vi "MainForceMeasurement.vi"() -> ()   [LabVIEW 2010]
uses:
  <vilib>/Instr/_visa.llb/VISA Flush IO Buffer Mask.ctl
  Variable globale 1.vi
  <vilib>/Instr/_visa.llb/VISA Configure Serial Port (Instr).vi
panel:
  out "Data":dbl[](array[numeric])
  out "Waveform Chart":dynamicdata(graph)
  in  "attente (ms)":u32=50
  in  "Temps échelon":i32=25
  out "Sor":string[][](array[string]) caption="Motor torque"
  out "Ent":string[][](array[string]) caption="Motor commande"
  out "Con_XYLeftTorque 2":cluster{"Y":dbl[], "Y":dbl[]}[](graph) caption="Sortie"
  out "Con_XYLeftTorque":cluster{"Y":dbl[], "Y":dbl[]}[](graph) caption="Commande"
  in  "Temps départ":i32=25
  out "tableau inversé 2":u8[](array[numeric])
  out "tableau inversé":i8[](array[numeric])
  out "error out 2":errorcluster caption="sortie d'erreur"
  in  "Type moteur":i32=139 min=0 max=255
  out "Float recu":sgl
  in  "Couple":sgl=25.45
  out "Iteration 3":i32
  out "Iteration reception":i32
  out "Iteration Envoi":i32
  out "Checksum calculé":i32
  out "Checksum reçu":i32
  out "Type de donnee (ID)":i32
  out "Byte Start ?":bool
  out "Retour 2":string
  in  "stop secu":bool
  in  "STOP":bool
  out "error out":errorcluster caption="sortie d'erreur"
  in  "baud rate (9600)":u32=9600 caption="débit en bauds (9600)"
  in  "Port Com":refnum<visa-resource-name>="COM7" caption="Nom de ressource VISA"
  # "Paramètre de l'envoi de l'échelon"
  # "Réception"
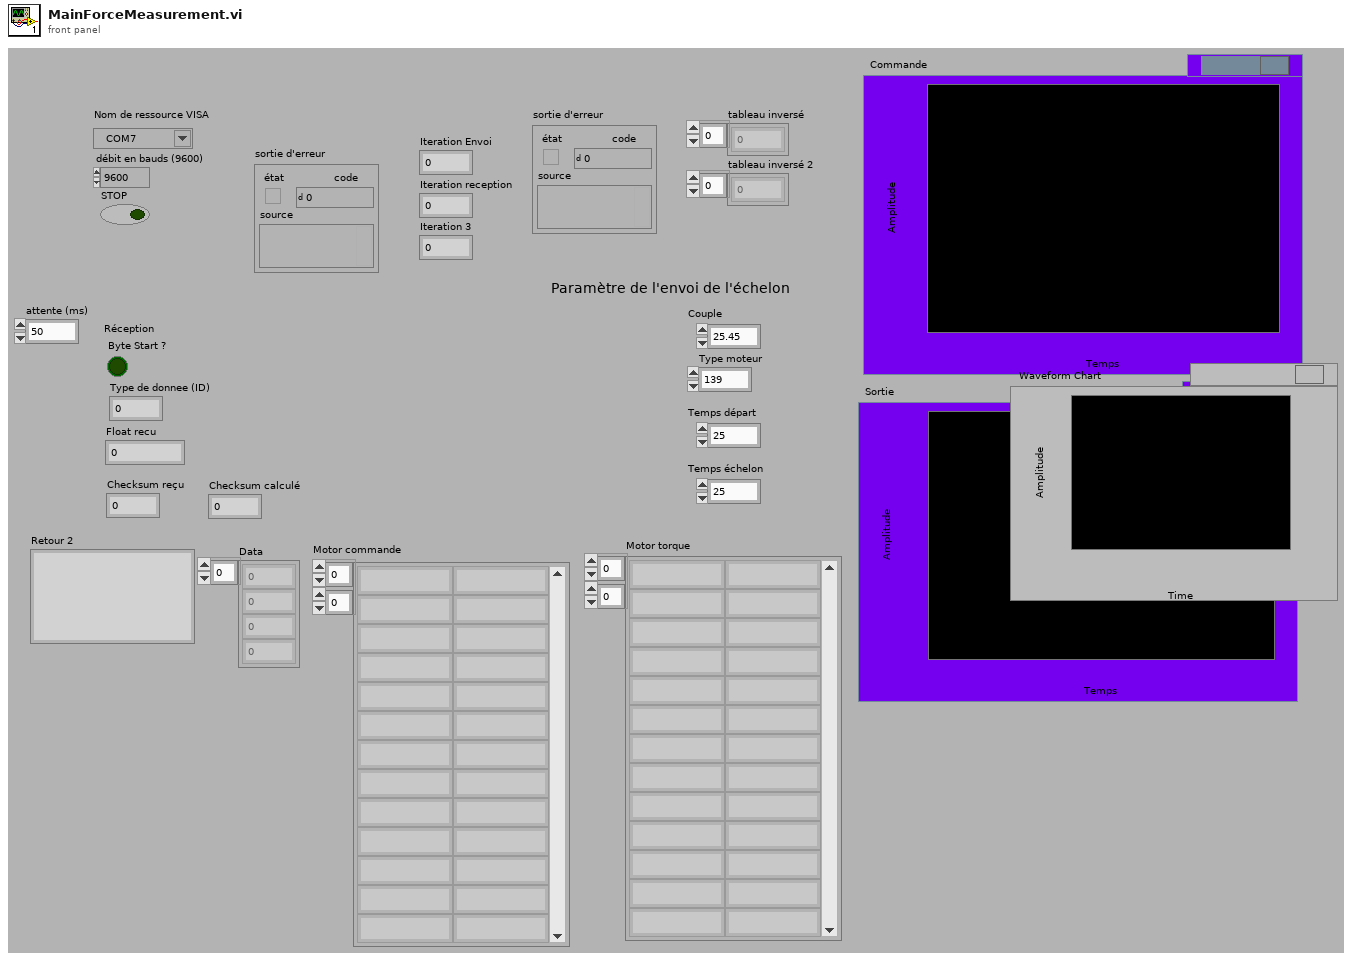
[diagram p1: front panel]
types:
  T1 = typedef "VISA Flush IO Buffer Mask.ctl" = u16
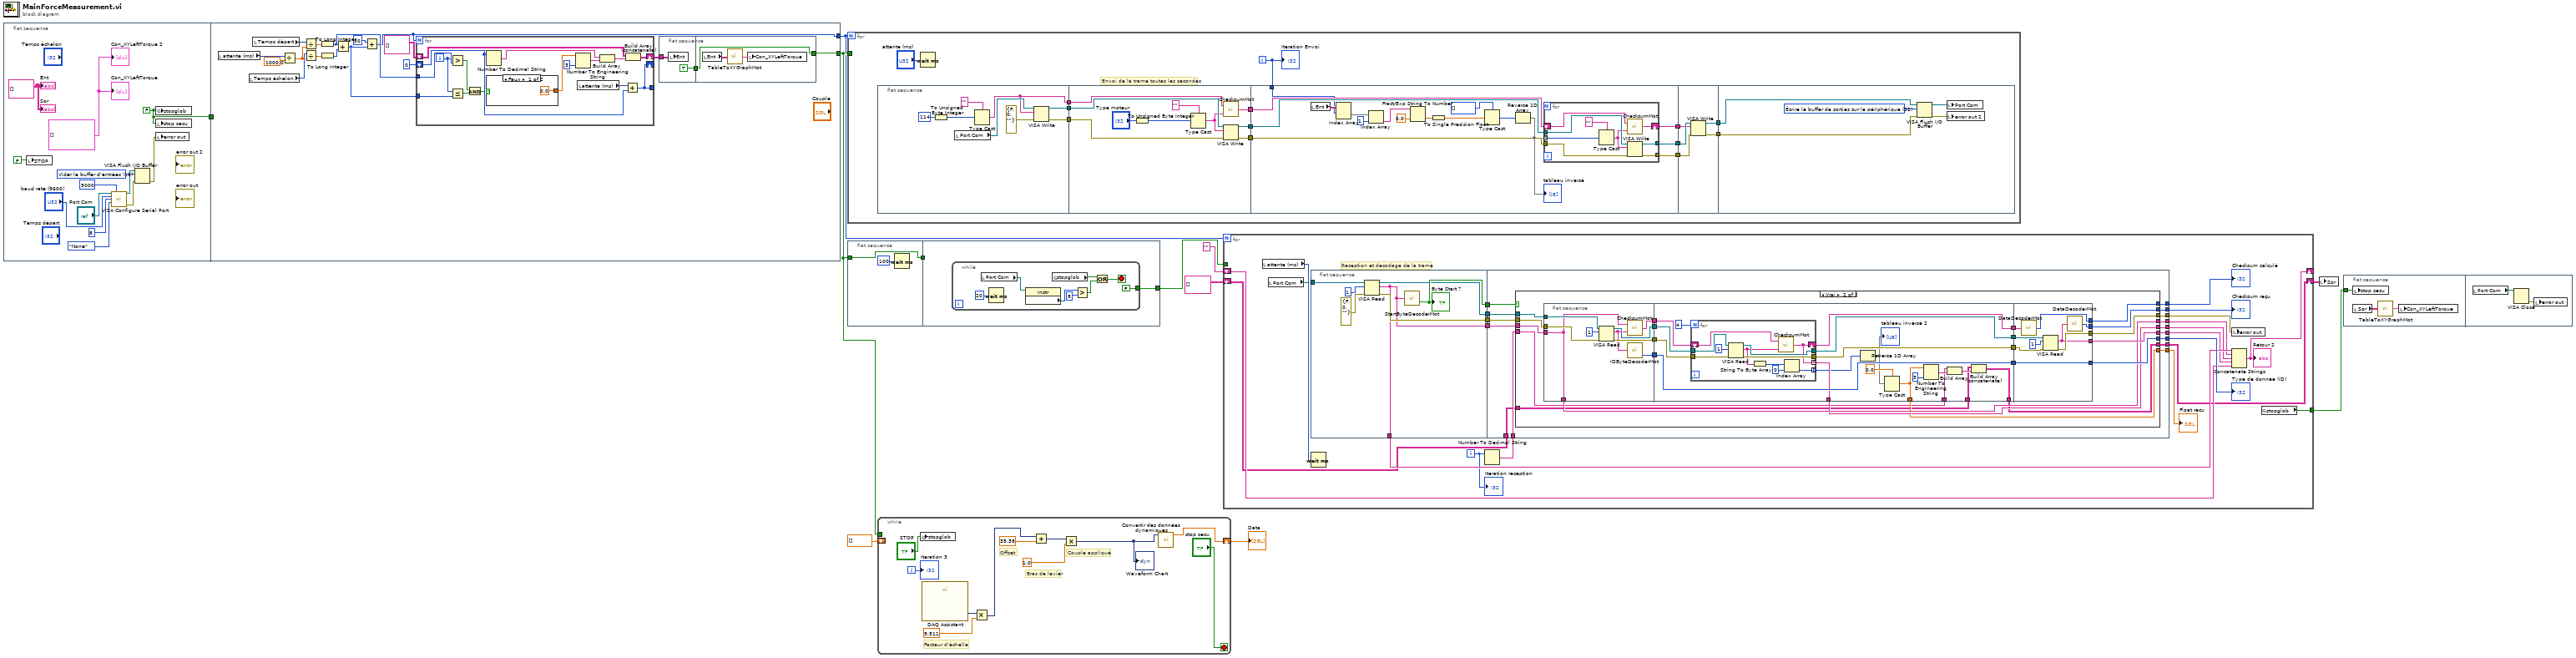
[diagram p0: block diagram]
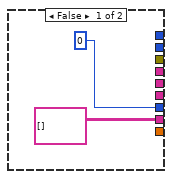
[diagram p2: hidden frame]
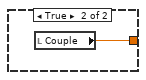
[diagram p3: hidden frame]
diagram:
  n1 = flat-sequence {
    tunnel: [w17] -> w7
    tunnel: [w33] -> w10
    tunnel: w7 -> [_]
    tunnel: [w28] -> w5
    frame #0 {
      w14 = cluster{"Y":dbl[], "Y":dbl[]}[] [] ("Con_XYLeftTorque 2")
      w13 = string[][] [] ("Con_MotorRightTorque")
      w17 = FALSE
      w19 = T1 16 items=["Vider le buffer d'entrées"=16, "Écrire le buffer de sorties sur le périphérique"=32, "Vider le buffer d'entrées (Pas d'E/S)"=64, "Vider le buffer de sorties"=128] ("Mask")
      n2 = local write "STOP"(FALSE) -> ()
      n3 = call-poly "VISA Configure Serial Port"("VISA resource name"="Port Com", "timeout (10sec)"=u32 5000, "baud rate (9600)"="baud rate (9600)", "data bits (8)"=u16 8, "parity (0:none)"=enum16{"None", "Odd", "Even", "Mark", "Space"}."None") -> ("VISA resource name out"=w16:refnum<visa-resource-name>, "error out"=w15:errorcluster)  [unwired: 9 in]
      n4 = VISA Flush I/O Buffer(VISA resource name=w16, mask (16)=w19, error in (no error)=w15) -> (error out=w18:errorcluster)  [unwired: 1 out]
      n5 = global write "Variable globale 1.vi" "stopglob"(w17) -> ()
      n6 = local write "stop secu"(w17) -> ()
      n7 = local write "error out"(w18) -> ()
      "Sor" <- w13
      "Con_XYLeftTorque" <- w14
      "Con_XYLeftTorque 2" <- w14
      "Ent" <- w13
    }
    frame #1 {
      n8 = local read "attente (ms)"() -> (w31:u32)
      n9 = local read "Temps échelon"() -> (w39:i32)
      n10 = local read "Temps départ"() -> (w41:i32)
      n11 = Divide(x=w31, y=sgl 1000.0) -> (x/y=w32:sgl)
      n12 = Divide(x=w41, y=w32) -> (x/y=w40:sgl)
      n13 = Divide(x=w39, y=w32) -> (x/y=w38:sgl)
      n14 = To Long Integer(number=w40) -> (32bit integer=w34:i32)
      n15 = To Long Integer(number=w38) -> (32bit integer=w37:i32)
      n16 = Add(x=w34, y=w37) -> (x+y=w26:i32)
      n17 = Add(x=50, y=w26) -> (x+y=w28:i32)
      n18 = for {
        N: w28 -> [_]
        shift-right: [w53] -> w29
        shift-left: string[][] [] ("Ent") -> [w54]
        shift-right: [w52] -> _
        shift-left: u32 0 -> [w62]
        tunnel: w34 -> [w60]
        tunnel: [w52] -> _
        tunnel: w26 -> [w50]
        i -> [w51]
        n19 = Greater?(x=w51, y=w60) -> (0:w49:bool)
        n20 = Less Or Equal?(x=w51, y=w50) -> (x <= y?=w48:bool)
        n21 = And(x=w49, y=w48) -> (x .and. y?=w47:bool)
        n22 = Number To Decimal String(number=w62) -> (decimal integer string=w59:string)  [unwired: 1 in]
        n23 = case shown="Faux" w47 {
          tunnel: [sgl 0.0 ("Couple") w64] -> w57
          frame False {
          }
          frame True {
            n24 = local read "Couple"() -> (w64:sgl)
          }
        }
        n25 = Number To Engineering String(2:i16 3 ("précision (6)"), 4:w57) -> (0:w58:string)  [unwired: 2 in]
        n26 = local read "attente (ms)"() -> (w61:u32)
        n27 = Build Array(w59, w58) -> (w55:string[])
        n28 = Add(x=w61, y=w62) -> (x+y=w52:u32)
        n29 = Build Array (concatenate)(w54, w55) -> (w53:string[][])
      }
      n30 = flat-sequence {
        tunnel: w29 -> [w42]
        tunnel: [TRUE] -> w25
        tunnel: [w46] -> w33
        tunnel: w25 -> [w46]
        frame #0 {
          n31 = local write "Ent"(w42) -> ()
        }
        frame #1 {
          n32 = local read "Ent"() -> (w44:string[][])
          n33 = call "TableToXYGraphMot.vi"("Input Table"=w44) -> ("XY Graph"=w45:cluster{"Y":dbl[], "Y":dbl[]}[])
          n34 = local write "Con_XYLeftTorque"(w45) -> ()
        }
      }
    }
  }
  n35 = for {
    N: w5 -> [_]
    tunnel: w10 -> [_]
    i -> [w65]
    # "Envoi de la trame toutes les secondes"
    n36 = flat-sequence {
      tunnel: [w82] -> w77
      tunnel: [w81] -> w76
      tunnel: [w80] -> w73
      tunnel: w77 -> [w95]
      tunnel: w76 -> [w94]
      tunnel: [w93] -> w75
      tunnel: [w92] -> w74
      tunnel: w73 -> [w91]
      tunnel: [w90] -> w72
      tunnel: w75 -> [w109]
      tunnel: w74 -> [w111]
      tunnel: w72 -> [w107]
      tunnel: [w110] -> w71
      tunnel: [w108] -> w70
      tunnel: [w106] -> w69
      tunnel: w65 -> [w102]
      tunnel: w71 -> [w126]
      tunnel: w70 -> [w125]
      tunnel: w69 -> [w124]
      tunnel: [w123] -> w67
      tunnel: [w122] -> w66
      tunnel: w67 -> [w131]
      tunnel: w66 -> [w130]
      frame #0 {
        n37 = To Unsigned Byte Integer(number=114) -> (unsigned 8bit integer=w79:u8)
        n38 = local read "Port Com"() -> (w85:refnum<visa-resource-name>)
        n39 = Type Cast(type="", x=w79) -> (*(type *) &x=w80:string)
        n40 = VISA Write(VISA resource name=w85, write buffer=w80, error in (no error)=errorcluster {"status"=FALSE, "code"=0, "source"=""} ("entrée d'erreur (pas d'erreur)")) -> (VISA resource name out=w82:refnum<visa-resource-name>, error out=w81:errorcluster)  [unwired: 1 out]
      }
      frame #1 {
        n41 = To Unsigned Byte Integer(number="Type moteur") -> (unsigned 8bit integer=w88:u8)
        n42 = Type Cast(type="", x=w88) -> (*(type *) &x=w86:string)
        n43 = call "ChecksumMot.vi"("Byte2"=w86, "Byte1"=w91) -> ("chaîne"=w90:string)
        n44 = VISA Write(VISA resource name=w95, write buffer=w86, error in (no error)=w94) -> (VISA resource name out=w92:refnum<visa-resource-name>, error out=w93:errorcluster)  [unwired: 1 out]
      }
      frame #2 {
        n45 = local read "Ent"() -> (w103:string[][])
        n46 = Index Array(array=w103, index (row)=w102) -> (element=w101:string[])  [unwired: 1 in]
        n47 = Index Array(array=w101, index=1 ("indice")) -> (element=w99:string)
        n48 = Fract/Exp String To Number(string=w99, default (0 dbl)=0.0 ("valeur par défaut (0 DBL)")) -> (number=w97:dbl)  [unwired: 2 in, 1 out]
        n49 = To Single Precision Float(number=w97) -> (single precision float=w96:sgl)
        n50 = Type Cast(type=i8[] [] ("tableau d'octets non signés"), x=w96) -> (*(type *) &x=w105:i8[])
        n51 = Reverse 1D Array(array=w105) -> (reversed array=w104:i8[])
        "tableau inversé" <- w104
        n52 = for {
          tunnel: w104 -> [w121] mode=indexing
          tunnel: w111 -> [w119]
          tunnel: [w118] -> w110
          tunnel: w109 -> [w117]
          tunnel: [w116] -> w108
          shift-right: [w113] -> w106
          shift-left: w107 -> [w115]
          n53 = Type Cast(type="", x=w121) -> (*(type *) &x=w114:string)
          n54 = call "ChecksumMot.vi"("Byte2"=w114, "Byte1"=w115) -> ("chaîne"=w113:string)
          n55 = VISA Write(VISA resource name=w119, write buffer=w114, error in (no error)=w117) -> (VISA resource name out=w118:refnum<visa-resource-name>, error out=w116:errorcluster)  [unwired: 1 out]
        }
      }
      frame #3 {
        n56 = VISA Write(VISA resource name=w126, write buffer=w124, error in (no error)=w125) -> (VISA resource name out=w123:refnum<visa-resource-name>, error out=w122:errorcluster)  [unwired: 1 out]
      }
      frame #4 {
        w127 = T1 32 items=["Vider le buffer d'entrées"=16, "Écrire le buffer de sorties sur le périphérique"=32, "Vider le buffer d'entrées (Pas d'E/S)"=64, "Vider le buffer de sorties"=128] ("Mask")
        n57 = VISA Flush I/O Buffer(VISA resource name=w131, mask (16)=w127, error in (no error)=w130) -> (VISA resource name out=w128:refnum<visa-resource-name>, error out=w129:errorcluster)
        n58 = local write "Port Com"(w128) -> ()
        n59 = local write "error out 2"(w129) -> ()
      }
    }
    n60 = Wait (ms)(milliseconds to wait="attente (ms)") -> ()  [unwired: 1 out]
    "Iteration Envoi" <- w65
  }
  n61 = flat-sequence {
    tunnel: w10 -> [w132]
    tunnel: [w132] -> w9
    tunnel: w9 -> [_]
    tunnel: [w134] -> w8
    frame #0 {
      n62 = Wait (ms)(milliseconds to wait=u32 100 ("attente (ms)")) -> ()  [unwired: 1 out]
    }
    frame #1 {
      n63 = while {
        tunnel: [FALSE] -> w134
        stop <- w141 stop-if-true
        n64 = local read "Port Com"() -> (w140:refnum<visa-resource-name>)
        n65 = Wait (ms)(milliseconds to wait=u32 20 ("attente (ms)")) -> ()  [unwired: 1 out]
        n66 = property class="Instr"(reference=w140) -> ("Serial Settings:Number of Bytes at Serial Port"=w139:u32)  [unwired: 1 in, 2 out]
        n67 = global read "Variable globale 1.vi" "stopglob"() -> (w142:bool)
        n68 = Greater?(x=w139, y=u32 8) -> (0:w137:bool)
        n69 = Or(x=w142, y=w137) -> (x .or. y?=w141:bool)
      }
    }
  }
  n70 = while {
    tunnel: w10 -> [_]
    shift-right: [w143] -> w2
    shift-left: dbl[] [] ("Array") -> [_]
    i -> [w151]
    stop <- "stop secu" stop-if-true
    # "Bras de levier"
    # "Couple appliqué"
    # "Offset"
    # "Facteur d'échelle"
    n71 = global write "Variable globale 1.vi" "stopglob"("STOP") -> ()
    n72 = call "DAQ Assistant"() -> ("data"=w145:dynamicdata)  [unwired: 17 in, 2 out]
    n73 = Multiply(x=w145, y=9.511) -> (x*y=w147:dynamicdata)
    n74 = Add(x=w147, y=35.38) -> (x+y=w149:dynamicdata)
    n75 = Multiply(x=w149, y=1.0) -> (x*y=w144:dynamicdata)
    "Waveform Chart" <- w144
    n76 = call "Convertir des données dynamiques"("Dynamic Data Type"=w144) -> ("Array"=w143:dbl[])  [unwired: 3 in]
    "Iteration 3" <- w151
  }
  "Data" <- w2
  n77 = for {
    N: w5 -> [_]
    shift-right: [w161] -> _
    shift-left: "" -> [w162]
    tunnel: w8 -> [_]
    tunnel: [w158] -> w6
    shift-right: [w154] -> w3
    shift-left: string[][] [] ("Sor") -> [w155]
    i -> [w157]
    # "Reception et decodage de la trame"
    n78 = local read "attente (ms)"() -> (w175:u32)
    n79 = local read "Port Com"() -> (w174:refnum<visa-resource-name>)
    n80 = flat-sequence {
      tunnel: w174 -> [w181]
      tunnel: [w180] -> w173
      tunnel: [w179] -> w172
      tunnel: [w178] -> w171
      tunnel: [w177] -> w169
      tunnel: [w177] -> w165
      tunnel: w173 -> [w197]
      tunnel: w172 -> [w196]
      tunnel: w171 -> [w195]
      tunnel: [w194] -> w170
      tunnel: w169 -> [w193]
      tunnel: [w192] -> w168
      tunnel: [w191] -> w167
      tunnel: [w190] -> w166
      tunnel: [w189] -> w164
      tunnel: [w188] -> w163
      tunnel: [w187] -> w160
      tunnel: [w186] -> w159
      tunnel: w156 -> [w185]
      tunnel: w155 -> [w184]
      tunnel: [w183] -> w154
      frame #0 {
        n81 = VISA Read(VISA resource name=w181, byte count=u32 1 ("nombre d'octets"), error in (no error)=errorcluster {"status"=FALSE, "code"=0, "source"=""} ("entrée d'erreur (pas d'erreur)")) -> (VISA resource name out=w179:refnum<visa-resource-name>, read buffer=w177:string, error out=w178:errorcluster)  [unwired: 1 out]
        n82 = call "StartByteDecoderMot.vi"("byte1"=w177) -> ("Byte Start ?"=w180:bool)  [unwired: 1 in]
        "Byte Start ?" <- w180
      }
      frame #1 {
        n83 = case shown="Vrai" w197 {
          tunnel: w196 -> [_ w221]
          tunnel: w195 -> [_ w220]
          tunnel: [0 ("Type de donnee (ID)") w219] -> w194
          tunnel: w193 -> [_ w214]
          tunnel: [_ w212] -> w192
          tunnel: [_ w211] -> w191
          tunnel: [_ w210] -> w190
          tunnel: [_ w209] -> w189
          tunnel: [_ w208] -> w188
          tunnel: [_ w205] -> w187
          tunnel: [_ w203] -> w186
          tunnel: w185 -> [_ w202]
          tunnel: w184 -> [_ w201]
          tunnel: [string[][] [] w200] -> w183
          frame False {
          }
          frame True {
            n84 = flat-sequence {
              tunnel: w221 -> [w230]
              tunnel: w220 -> [w229]
              tunnel: [w227] -> w218
              tunnel: [w226] -> w217
              tunnel: [w225] -> w216
              tunnel: w214 -> [w222]
              tunnel: [w223] -> w213
              tunnel: [w222] -> w209
              tunnel: w218 -> [w249]
              tunnel: w217 -> [w248]
              tunnel: w216 -> [w245]
              tunnel: [w249] -> w215
              tunnel: w213 -> [w243]
              tunnel: [w247] -> w207
              tunnel: [w246] -> w206
              tunnel: [w237] -> w205
              tunnel: [w242] -> w204
              tunnel: [w240] -> w203
              tunnel: w202 -> [w234]
              tunnel: w201 -> [w232]
              tunnel: [w231] -> w200
              tunnel: [w269] -> w219
              tunnel: w215 -> [w269]
              tunnel: [w267] -> w212
              tunnel: [w266] -> w211
              tunnel: [w265] -> w210
              tunnel: [w264] -> w208
              tunnel: w207 -> [w263]
              tunnel: w206 -> [w262]
              tunnel: w204 -> [w261]
              frame #0 {
                n85 = VISA Read(VISA resource name=w230, byte count=u32 1 ("nombre d'octets"), error in (no error)=w229) -> (VISA resource name out=w226:refnum<visa-resource-name>, read buffer=w224:string, error out=w225:errorcluster)  [unwired: 1 out]
                n86 = call "ChecksumMot.vi"("Byte2"=w224, "Byte1"=w222) -> ("chaîne"=w223:string)
                n87 = call "IDByteDecoderMot.vi"("byte1"=w224) -> ("Type de donnee (ID)"=w227:i32)  [unwired: 2 out]
              }
              frame #1 {
                n88 = for {
                  N: 4 -> [_]
                  tunnel: w248 -> [w259]
                  tunnel: [w258] -> w247
                  tunnel: [w257] -> w246
                  tunnel: w245 -> [w256]
                  tunnel: [w253] -> w239 mode=indexing
                  shift-right: [w250] -> w242
                  shift-left: w243 -> [w252]
                  tunnel: [w250] -> w240 mode=indexing
                  n89 = VISA Read(VISA resource name=w259, byte count=u32 1 ("nombre d'octets"), error in (no error)=w256) -> (VISA resource name out=w258:refnum<visa-resource-name>, read buffer=w251:string, error out=w257:errorcluster)  [unwired: 1 out]
                  n90 = String To Byte Array(string=w251) -> (unsigned byte array=w255:u8[])
                  n91 = call "ChecksumMot.vi"("Byte2"=w251, "Byte1"=w252) -> ("chaîne"=w250:string)
                  n92 = Index Array(array=w255, index=0 ("indice")) -> (element=w253:u8)
                }
                n93 = Reverse 1D Array(array=w239) -> (reversed array=w238:u8[])
                "tableau inversé 2" <- w238
                n94 = Type Cast(type=sgl 0.0, x=w238) -> (*(type *) &x=w237:sgl)
                n95 = Number To Engineering String(2:i16 3 ("précision (6)"), 4:w237) -> (0:w235:string)  [unwired: 2 in]
                n96 = Build Array(w234, w235) -> (w233:string[])
                n97 = Build Array (concatenate)(w232, w233) -> (w231:string[][])
              }
              frame #2 {
                n98 = call "DataDecoderMot.vi"("byte1"=w261) -> ("Data"=w267:i32)
                n99 = VISA Read(VISA resource name=w263, byte count=u32 1 ("nombre d'octets"), error in (no error)=w262) -> (read buffer=w264:string, error out=w265:errorcluster)  [unwired: 2 out]
                n100 = call "DataDecoderMot.vi"("byte1"=w264) -> ("Data"=w266:i32)
              }
            }
          }
        }
      }
    }
    n101 = Wait (ms)(milliseconds to wait=w175) -> ()  [unwired: 1 out]
    n102 = Number To Decimal String(number=w157) -> (decimal integer string=w156:string)  [unwired: 1 in]
    n103 = local write "error out"(w166) -> ()
    n104 = Concatenate Strings(w165, w164, w159, w163, w162) -> (w161:string)
    "Retour 2" <- w161
    n105 = global read "Variable globale 1.vi" "stopglob"() -> (w158:bool)
    "Type de donnee (ID)" <- w170
    "Checksum reçu" <- w167
    "Checksum calculé" <- w168
    "Iteration reception" <- w157
    "Float recu" <- w160
  }
  n106 = local write "Sor"(w3) -> ()
  n107 = flat-sequence {
    tunnel: w6 -> [w272]
    frame #0 {
      n108 = local write "stop secu"(w272) -> ()
      n109 = local read "Sor"() -> (w271:string[][])
      n110 = call "TableToXYGraphMot.vi"("Input Table"=w271) -> ("XY Graph"=w270:cluster{"Y":dbl[], "Y":dbl[]}[])
      n111 = local write "Con_XYLeftTorque"(w270) -> ()
    }
    frame #1 {
      n112 = local read "Port Com"() -> (w274:refnum<visa-resource-name>)
      n113 = VISA Close(VISA resource name=w274) -> (error out=w273:errorcluster)  [unwired: 1 in]
      n114 = local write "error out"(w273) -> ()
    }
  }
